vi "Shift Correction Array (Latency Compensation).vi"(10 "Correction Shift (mm)":ext, 11 "Compensation In (%)":cluster{dbl[], dbl[]}) -> (3 "Compensation Out (%)":cluster{ext[], dbl[]})   [LabVIEW 2016]
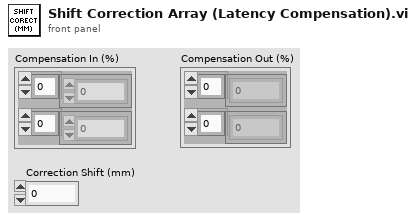
[diagram p1: front panel]
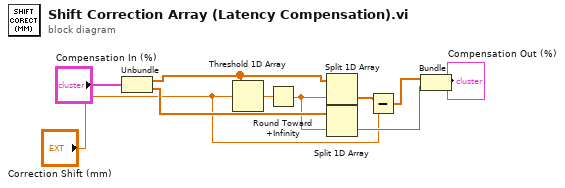
[diagram p0: block diagram]
diagram:
  n1 = Unbundle("Compensation In (%)") -> (w6:dbl[], w7:dbl[])
  n2 = Threshold 1D Array(2:"Correction Shift (mm)", 3:w6) -> (0:w2:dbl)  [unwired: 1 in]
  n3 = Round Toward +Infinity(x=w2) -> (ceil(x): smallest int >= x=w1:dbl)
  n4 = Split 1D Array(array=w6, index=w1) -> (second subarray=w3:dbl[])  [unwired: 1 out]
  n5 = Split 1D Array(array=w7, index=w1) -> (second subarray=w9:dbl[])  [unwired: 1 out]
  n6 = Subtract(x=w3, y="Correction Shift (mm)") -> (x-y=w8:ext[])
  n7 = Bundle(w8, w9) -> (→"Compensation Out (%)":cluster{ext[], dbl[]})  [unwired: 1 in]
